vi "FPGA Co-Wound Test.vi"() -> ()   [LabVIEW 2018]
doc: "Author: Scott Hannahs <sth@magnet.fsu.edu>\nCopyright 2018 Florida State University, All rights reserved."
uses:
  <vilib>/eio/EIONode/EIONode.xnode
  <vilib>/rvi/eio/common/nirviEmuTemplateMethod_errors.vi
  SCH Data Controls/Digitizer State Enum.ctl
  SCH Data Controls/SCH Data 2 RT.ctl
  SCH Data Controls/SCH Int Data with Pressure.ctl
  SCH Data Controls/SCH Raw Int Data.ctl
  <vilib>/rvi/FXPMathLib/FxpInterpret/XNode/nifxpmath_Interpret.xnode
  <vilib>/rvi/DataTransferAndStorage/Container/XNode/niFpgaContainer.xnode
  <vilib>/rvi/interface/RandomDataEmulation/nirviRandomDataFpgaReadWriteTemplate.vi
  <vilib>/rvi/FIFO/Fifo_Resource/nirvififoEmulationWrite.vi
  SCH Scaling Controls/SCH Pressure Offset.ctl
  SCH Scaling Controls/SCH Pressure Offset Array.ctl
  SCH Scaling Controls/SCH Dump Resistor Scale Factor.ctl
  SCH Scaling Controls/SCH Joint Scale Factor.ctl
  SCH Scaling Controls/SCH Joint Scale Factor Array.ctl
  SCH Scaling Controls/SCH SC Bus Scale Factor.ctl
  SCH Scaling Controls/SCH SC Bus Scale Factor Array.ctl
  SCH Scaling Controls/SCH CoWound Scale Factor.ctl
  SCH Scaling Controls/SCH Scale Factor.ctl
  SCH Scaling Controls/SCH Scale Factor Array.ctl
  SCH Data Controls/SCH Data 2 RT Array.ctl
  Init Coil Calibration/FPGA Magnet Config.ctl
panel:
  in  "Magnet Configuration Data":T1={"#Coils"=4, "Coil Inductances"=[0.10000002384185791, 0.3999999761581421, 0.6000000238418579, 1.199999988079071], "Max Coil Currents"=[19.899999976158142, 19.899999976158142, 19.899999976158142, 19.899999976158142], "Max Coil Volt Dev"=[1.800000011920929, 2.100000023841858, 3.100000023841858, 2.600000023841858], "Coil A Coefficients"=[0.8209999799728394, 0.00010001659393310547, 5.960464477539063e-08], "Coil B Coefficients"=[0.8999999761581421, 0.00019997358322143555, 2.9802322387695312e-06], "Coil C Coefficients"=[1.100000023841858, 0.0, 0.0], "Coil D Coefficients"=[1.0, 0.0009999871253967285, 0.0], "Max Coil Temp"=[100.0, 80.0, 80.0, 60.0], " Pressure Range"=[29.30000001192093, 32.30000001192093], "Temp Coef"=[0.0031999945640563965, 0.0031999945640563965, 0.0029000043869018555, 0.004100024700164795], "Offsets"=[0.0, 0.0, -5.0, -5.0, 0.0, 0.0, 0.0, 0.0, 0.0, 0.0, 0.0, 0.0, 0.0, 0.0, 0.0], "Scale Factors"=[20.0, 20.0, 4.2670000195503235, 4.269999980926514, 2.0, 1.0, 1.0, 1.0, 1.0, 1.0, -2.0, 30.08600002527237, 29.861999988555908, 35.50199997425079, 35.56999999284744]} {"Coil D Coefficients" format="%_6g"; "Coil C Coefficients" format="%_6g"; "Coil B Coefficients" format="%_6g"; "Scale Factors" format="%_5g"; "Offsets" format="%_5g"; "Temp Coef" format="%_6g"; "Max Coil Temp" format="%_6g"; "Max Coil Volt Dev" format="%_6g"; "Max Coil Currents" format="%_6g"; "Coil Inductances" format="%_6g"; "Pressure Range" format="%_6g"; "Coil A Coefficients" format="%_6g"}
  in  "Input Select":T3(ring)
  in  "Inject frequency (Hz)":fxp<+,32,16>
  in  "Inject Offset":fxp<+/-,16,5> format="%.3g"
  in  "Inject Channel":i32=1
  out "Scale":T4
  out "Calibrate Index":i16
  out "Offset":T4
  out "Main Index":i32
  in  "Reset":bool
  out "DAQ Loop WDT":bool
  out "Filt Data":T5=[0.0, 0.0, 0.0, 0.0, 0.0, 0.0, 0.0, 0.0, 0.0, 0.0, 0.0, 0.0, 0.0, 0.0, 0.0, 0.0, 0.0, 0.0, 0.0, 0.0, 0.0, 0.0, 0.0, 0.0, 0.0, 0.0, 0.0, 0.0, 0.0, 0.0, 0.0, 0.9999999701976776, 0.0, 0.0, -1.0, 0.9999999701976776, -1.0, -1.0, 0.9971923828125, 0.0, 0.0, 0.0, 0.0, 0.0, 0.0, -1.0, 0.0, 0.0, 0.0, 0.0, 0.0, 0.0, 0.0, 0.0] format="%_6g"
  out "Filt Data 2":T5 format="%_6g"
  in  "Layer Scale Factors":T6=[3.0, 3.0, 3.0, 3.0, 3.0, 3.0, 3.0, 3.0, 3.0, 3.0, 3.0, 3.0, 3.0, 3.0, 3.0, 3.0, 3.0, 3.0]
  in  "Co-Wound Scale Factor":T8=200.0
  in  "SC Bus Scale":T9=[0.0009765326976776123, 0.0009765326976776123, 0.0009765326976776123, 0.0009765326976776123, 0.0009765326976776123, 0.0009765326976776123]
  in  "Joint Scale Factors":T11=[1.0013580322265625e-05, 1.0013580322265625e-05, 1.0013580322265625e-05, 1.0013580322265625e-05, 1.0013580322265625e-05, 1.0013580322265625e-05, 1.0013580322265625e-05, 1.0013580322265625e-05]
  in  "DAQ Cycle Ticks":u32=4096
  out "uSec/Cycle":u32
  in  "Ln2 Filter Size":i16=10
  in  "Dump Resistor Scale Factor":T13=200.0
  out "Dump Resistor Voltage":T2 format="%_6g"
  in  "Pressure Offsets":T14=[-8.5, -8.5]
  out "Data Size":i32
  out "Timed Out? FIFO2RT Filter":bool
  out "Timed Out? FIFO Raw":bool
  in  "Pressure Scale Factor":T2[](array[typedef])=[1.723690003156662, 1.723690003156662, 1.723690003156662, 1.723690003156662] format="%_6g"
  in  "stop 2":bool
  out "Timed Out? FIFO2RT Raw":bool
  in  "stop":bool
  # "mH"
  # "kA"
  # "V"
  # "mOhm"
  # "mOhm"
  # "mOhm"
  # "mOhm"
  # "Deg C"
  # "bar"
  # "1/Deg C"
  # "Tin"
  # "Tout"
  # "Pin"
  # "Pout"
  # "I"
  # "WDTin"
  # "PSEnb"
  # "CellFLT"
  # "WDTout"
  # "BTFlt"
  # "BTvolt"
  # "Va"
  # "Vb"
  # "Vc"
  # "Vd"
  # "Tin"
  # "Tout"
  # "Pin"
  # "Pout"
  # "I"
  # "WDTin"
  # "PSEnb"
  # "CellFLT"
  # "WDTout"
  # "BTFlt"
  # "BTvolt"
  # "Va"
  # "Vb"
  # "Vc"
  # "Vd"
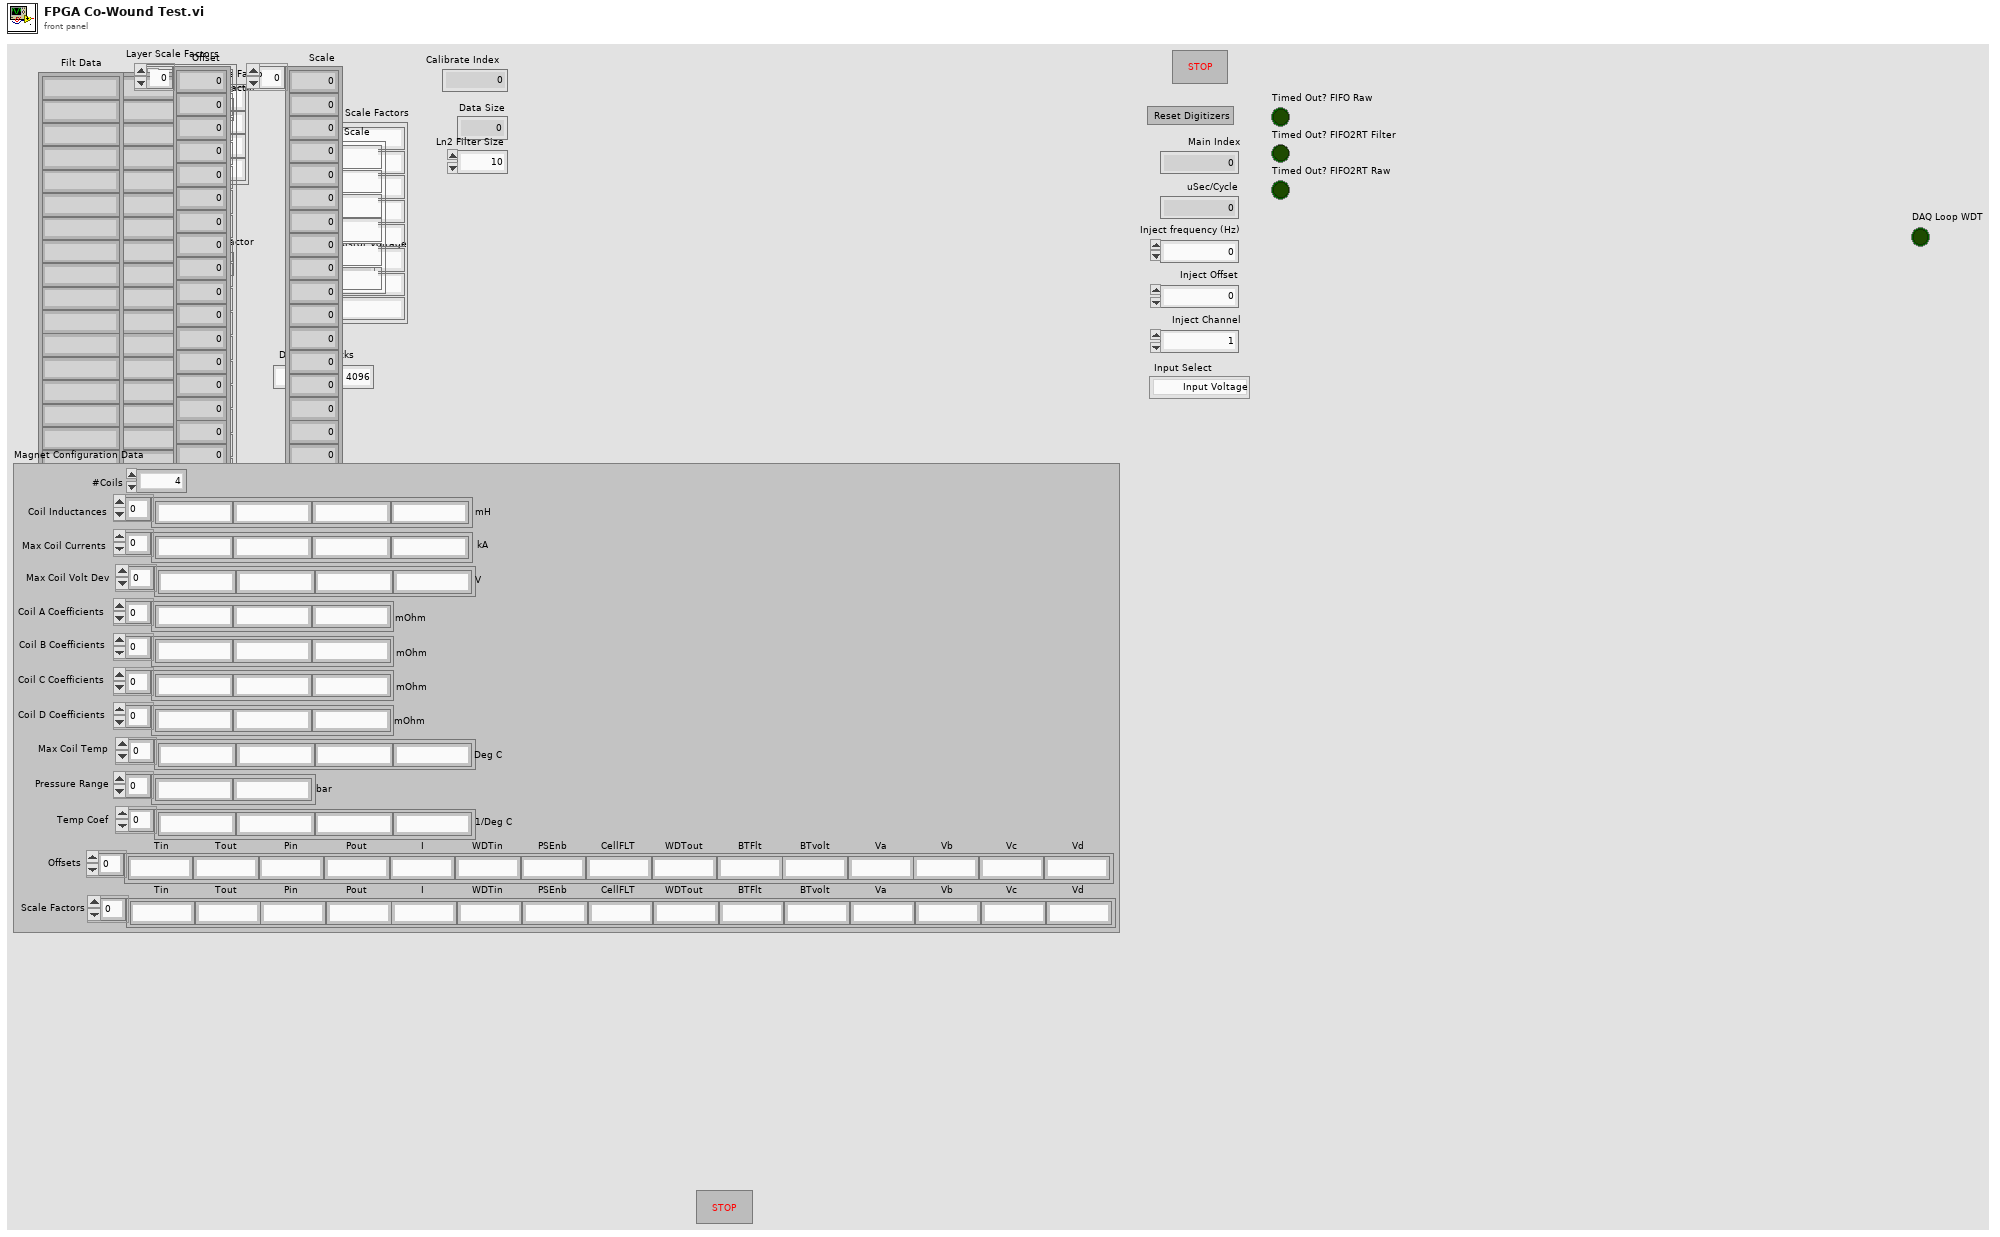
[diagram p1: front panel]
types:
  T1 = typedef "FPGA Magnet Config.ctl" = cluster{"#Coils":u32, "Coil Inductances":T2[], "Max Coil Currents":T2[], "Max Coil Volt Dev":T2[], "Coil A Coefficients":T2[], "Coil B Coefficients":T2[], "Coil C Coefficients":T2[], "Coil D Coefficients":T2[], "Max Coil Temp":T2[], " Pressure Range":T2[], "Temp Coef":T2[], "Offsets":T2[], "Scale Factors":T2[]}
  T2 = typedef "SCH Data 2 RT.ctl" = fxp<+/-,38,12>
  T3 = enum16{"Input Voltage", "Zero Voltage", "Calibrate Voltage"}
  T4 = typedef "SCH Raw Int Data.ctl" = i16[]
  T5 = typedef "SCH Data 2 RT Array.ctl" = T2[]
  T6 = typedef "SCH Scale Factor Array.ctl" = T7[]
  T7 = typedef "SCH Scale Factor.ctl" = fxp<+/-,16,6>
  T8 = typedef "SCH CoWound Scale Factor.ctl" = fxp<+/-,16,12>
  T9 = typedef "SCH SC Bus Scale Factor Array.ctl" = T10[]
  T10 = typedef "SCH SC Bus Scale Factor.ctl" = fxp<+/-,38,12>
  T11 = typedef "SCH Joint Scale Factor Array.ctl" = T12[]
  T12 = typedef "SCH Joint Scale Factor.ctl" = fxp<+/-,38,12>
  T13 = typedef "SCH Dump Resistor Scale Factor.ctl" = fxp<+/-,16,12>
  T14 = typedef "SCH Pressure Offset Array.ctl" = T15[]
  T15 = typedef "SCH Pressure Offset.ctl" = fxp<+/-,16,5>
  T16 = typedef "Digitizer State Enum.ctl" = enum16{"Reset", "StartCnvt"}
  T17 = typedef "SCH Int Data with Pressure.ctl" = fxp<+/-,19,5>[]
  T18 = typedef "SCH All FXP Data.ctl" = fxp<+/-,19,5>[]
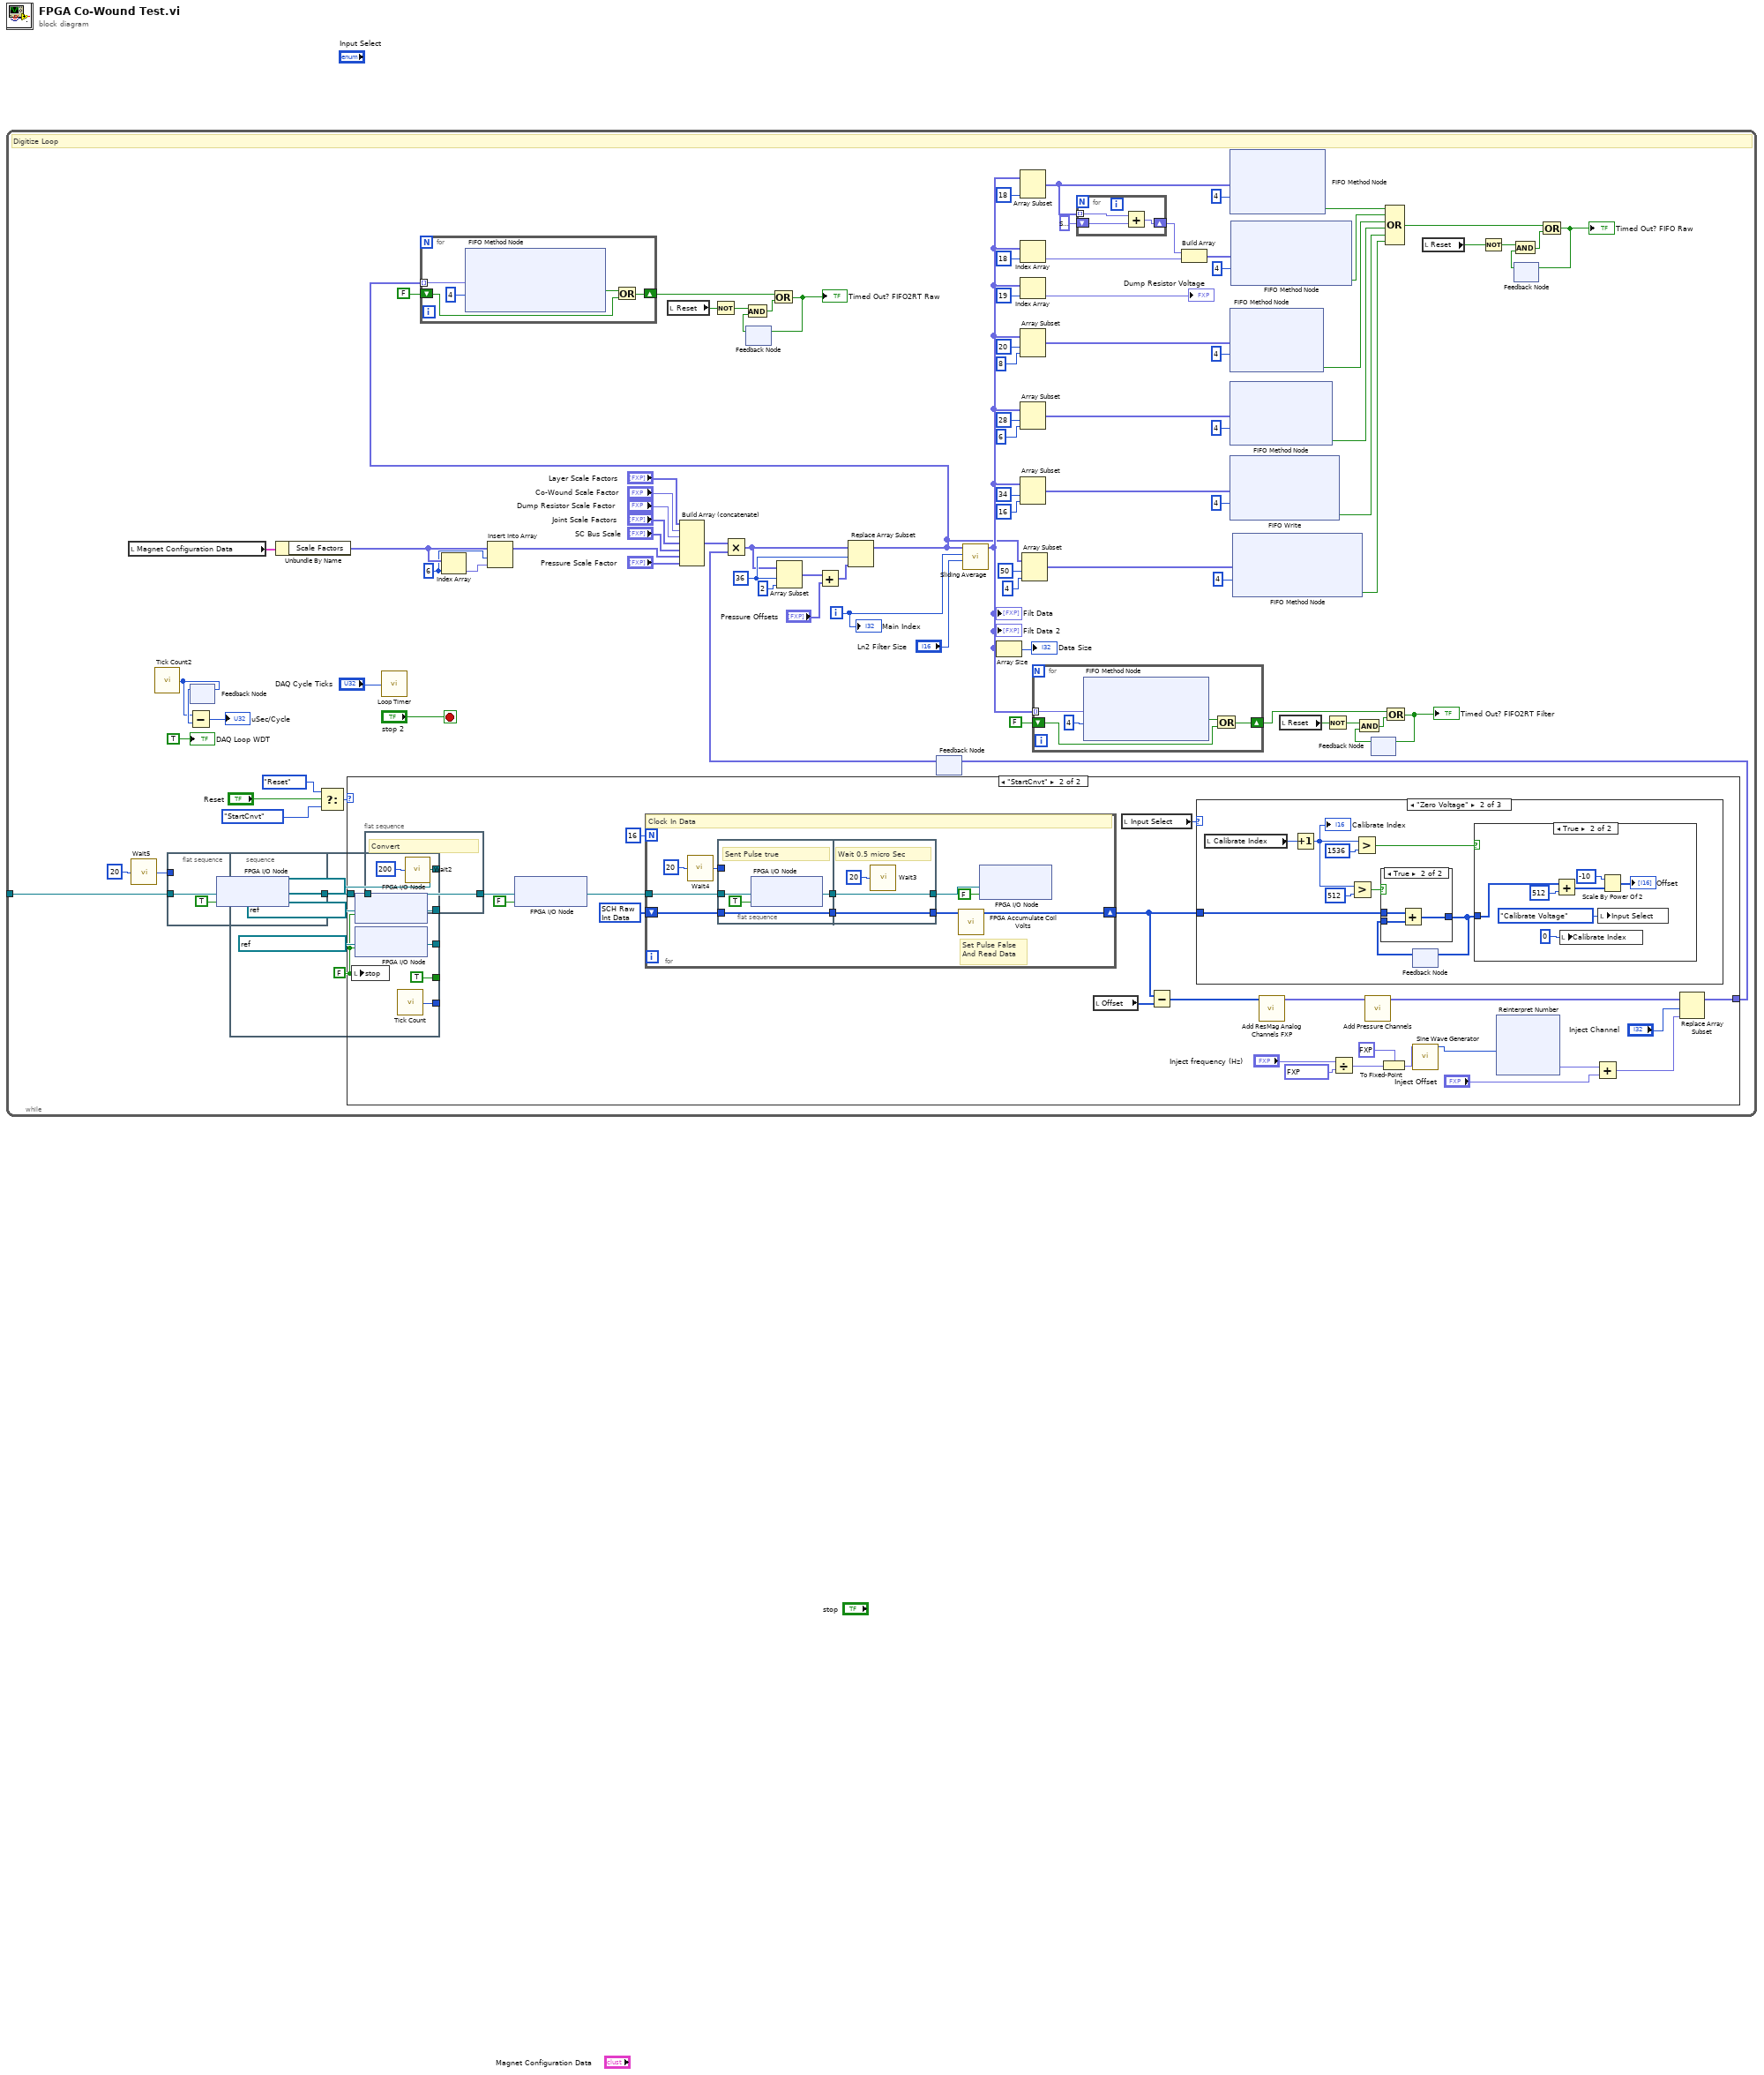
[diagram p0: block diagram]
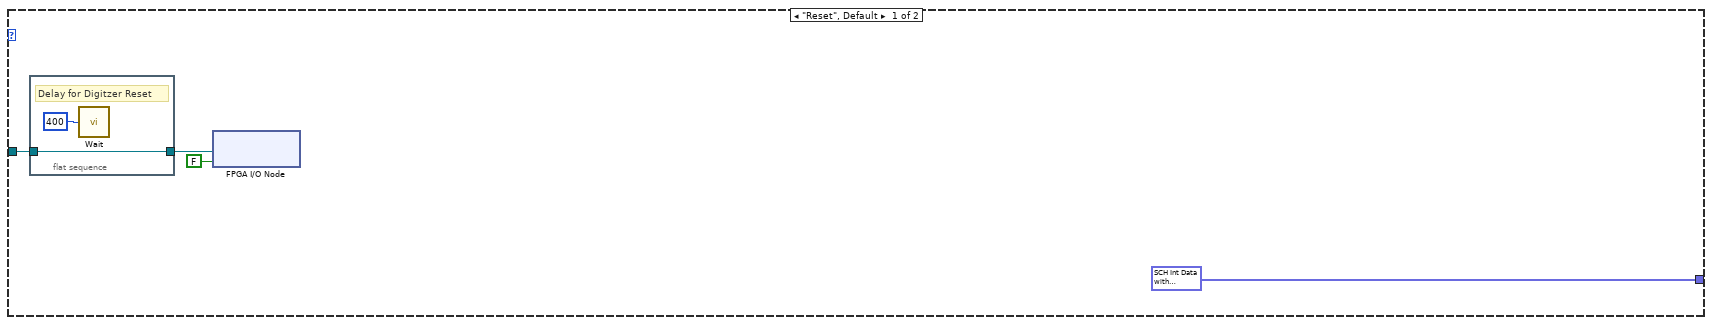
[diagram p2: hidden frame]
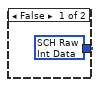
[diagram p5: hidden frame]
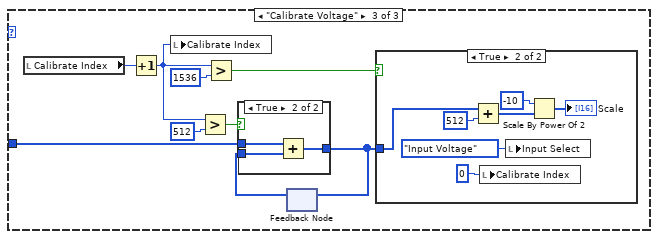
[diagram p6: hidden frame]
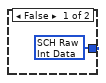
[diagram p8: hidden frame]
diagram:
  n1 = while {
    tunnel: _ -> [w87]
    i -> [w58]
    stop <- "stop 2" stop-if-true
    w29 = 6 ("index")
    w62 = 36 ("index")
    # "Digitize Loop"
    n2 = local read "Magnet Configuration Data"() -> (w76:T1)
    n3 = call "Wait5"("Count(Ticks)"=u32 20 ("Count(uSec)")) -> ("Tick Count(Ticks)"=w88:u32)
    n4 = call "Tick Count2"() -> ("Tick Count(uSec)"=w71:u32)
    n5 = flat-sequence {
      tunnel: w88 -> [_]
      tunnel: w87 -> [w107]
      tunnel: [w106] -> w86
      frame #0 {
        n6 = xnode "FPGA I/O Node"("I/O Item"=TRUE ("Connector0/DIO0"), "FPGA I/O In"=w107) -> ("FPGA I/O Out"=w106:refnum<k21>)
      }
    }
    n7 = feedback #1() -> (w72:u32)  [unwired: 1 in]
    n8 = Subtract(x=w71, y=w72) -> (x-y=→"uSec/Cycle":u32)
    n9 = feedback-in #1(w71) -> ()
    n10 = Unbundle By Name(w76) -> ("Scale Factors"=w30:T2[])
    n11 = Select(t=Digitizer_State_Enum."Reset", s="Reset", f=Digitizer_State_Enum."StartCnvt" ("t")) -> (s? t:f=w90:T16)
    n12 = case shown="\"StartCnvt\"" w90 {
      tunnel: w86 -> [w110 w135]
      tunnel: [T17 [0.0, 0.0, 0.0, 0.0, 0.0, 0.0, 0.0, 0.0, 0.0, 0.0, 0.0, 0.0, 0.0, 0.0, 0.0, 0.0, 0.0, 0.0, 0.0, 0.0, 0.0, 0.0, 0.0, 0.0, 0.0, 0.0, 0.0, 0.0, 0.0, 0.0, 0.0, 0.0, 0.0, 0.0, 0.0, 0.0, 0.0, 0.0, 0.0, 0.0, 0.0, 0.0, 0.0, 0.0, 0.0, 0.0, 0.0, 0.0, 0.0, 0.0, 0.0, 0.0, 0.0, 0.0] ("Array") w130] -> w73
      frame "Reset", Default {
        n13 = flat-sequence {
          tunnel: [w114] -> w111
          tunnel: w110 -> [w114]
          frame #0 {
            # "Delay for Digitzer Reset"
            n14 = call "Wait"("Count(Ticks)"=u32 400 ("Count(uSec)")) -> ()  [unwired: 1 out]
          }
        }
        n15 = xnode "FPGA I/O Node"("I/O Item"=FALSE ("Connector0/DIO0"), "FPGA I/O In"=w111) -> ()  [unwired: 1 out]
      }
      frame "StartCnvt" {
        n16 = flat-sequence {
          tunnel: [w195] -> w134
          tunnel: w135 -> [w195]
          frame #0 {
            # "Convert"
            n17 = call "Wait2"("Count(Ticks)"=u32 200 ("Count(uSec)")) -> ()  [unwired: 1 out]
          }
        }
        n18 = xnode "FPGA I/O Node"("I/O Item"=FALSE ("Connector0/DIO0"), "FPGA I/O In"=w134) -> ("FPGA I/O Out"=w136:refnum<k21>)
        n19 = for {
          N: 16 -> [_]
          shift-right: [w178] -> w115
          shift-left: T4 [0, 0, 0, 0, 0, 0, 0, 0, 0, 0, 0, 0, 0, 0, 0, 0, 0, 0, 0, 0, 0, 0, 0, 0, 0, 0, 0, 0, 0, 0, 0, 0, 0, 0, 0, 0, 0, 0] -> [w181]
          tunnel: w136 -> [w182]
          # "Set Pulse False\nAnd Read Data"
          # "Clock In Data"
          n20 = call "Wait4"("Count(Ticks)"=u32 20 ("Count(uSec)")) -> ("Tick Count(Ticks)"=w185:u32)
          n21 = flat-sequence {
            tunnel: w185 -> [_]
            tunnel: w182 -> [w190]
            tunnel: [w189] -> w187
            tunnel: w181 -> [w188]
            tunnel: [w188] -> w180
            tunnel: [w194] -> w184
            tunnel: w187 -> [w194]
            tunnel: [w192] -> w179
            tunnel: w180 -> [w192]
            frame #0 {
              # "Sent Pulse true"
              n22 = xnode "FPGA I/O Node"("I/O Item"=TRUE ("Connector0/DIO0"), "FPGA I/O In"=w190) -> ("FPGA I/O Out"=w189:refnum<k21>)
            }
            frame #1 {
              # "Wait 0.5 micro Sec"
              n23 = call "Wait3"("Count(Ticks)"=u32 20 ("Count(uSec)")) -> ()  [unwired: 1 out]
            }
          }
          n24 = call "FPGA Accumulate Coil Volts.vi"("Data Array In"=w179) -> ("Data Array Out"=w178:T4)  [unwired: 10 in]
          n25 = xnode "FPGA I/O Node"("I/O Item"=FALSE ("Connector0/DIO0"), "FPGA I/O In"=w184) -> ()  [unwired: 1 in, 2 out]
        }
        n26 = local read "Offset"() -> (w122:T4)
        n27 = local read "Input Select"() -> (w121:T3)
        n28 = Subtract(x=w115, y=w122) -> (x-y=w120:T4)
        n29 = case shown="\"Zero Voltage\"" w121 {
          tunnel: w115 -> [_ w143 w163]
          frame "Input Voltage", Default {
          }
          frame "Zero Voltage" {
            n30 = local read "Calibrate Index"() -> (w145:i16)
            n31 = Increment(x=w145) -> (x+1=w138:i16)
            "Calibrate Index" <- w138
            n32 = Greater?(x=w138, y=i16 512) -> (0:w144:bool)
            n33 = Greater?(x=w138, y=i16 1536) -> (0:w141:bool)
            n34 = feedback #2() -> (w139:i32[])  [unwired: 1 in]
            n35 = case shown="True" w144 {
              tunnel: w143 -> [_ w157]
              tunnel: [T4 [0, 0, 0, 0, 0, 0, 0, 0, 0, 0, 0, 0, 0, 0, 0, 0, 0, 0, 0, 0, 0, 0, 0, 0, 0, 0, 0, 0, 0, 0, 0, 0, 0, 0, 0, 0, 0, 0] ("Scale") w156] -> w140
              tunnel: w139 -> [_ w155]
              frame False {
              }
              frame True {
                n36 = Add(x=w157, y=w155) -> (x+y=w156:i32[])
              }
            }
            n37 = feedback-in #2(w140) -> ()
            n38 = case shown="True" w141 {
              tunnel: w140 -> [_ w152]
              frame False {
              }
              frame True {
                n39 = Add(x=w152, y=512 ("n")) -> (x+y=w148:i32[])
                n40 = local write "Calibrate Index"(i16 0 ("Calibrate Index")) -> ()
                n41 = local write "Input Select"(T3."Calibrate Voltage" ("Input Select")) -> ()
                n42 = Scale By Power Of 2(n=i16 -10, x=w148) -> (x*2^n=→"Offset":i32[])
              }
            }
          }
          frame "Calibrate Voltage" {
            n43 = local read "Calibrate Index"() -> (w165:i16)
            n44 = Increment(x=w165) -> (x+1=w158:i16)
            n45 = local write "Calibrate Index"(w158) -> ()
            n46 = Greater?(x=w158, y=i16 512) -> (0:w164:bool)
            n47 = Greater?(x=w158, y=i16 1536) -> (0:w161:bool)
            n48 = feedback #3() -> (w159:i32[])  [unwired: 1 in]
            n49 = case shown="True" w164 {
              tunnel: w163 -> [_ w177]
              tunnel: [T4 [0, 0, 0, 0, 0, 0, 0, 0, 0, 0, 0, 0, 0, 0, 0, 0, 0, 0, 0, 0, 0, 0, 0, 0, 0, 0, 0, 0, 0, 0, 0, 0, 0, 0, 0, 0, 0, 0] ("Scale") w176] -> w160
              tunnel: w159 -> [_ w175]
              frame False {
              }
              frame True {
                n50 = Add(x=w177, y=w175) -> (x+y=w176:i32[])
              }
            }
            n51 = feedback-in #3(w160) -> ()
            n52 = case shown="True" w161 {
              tunnel: w160 -> [_ w172]
              frame False {
              }
              frame True {
                n53 = Add(x=w172, y=512 ("n")) -> (x+y=w168:i32[])
                n54 = local write "Calibrate Index"(i16 0 ("Calibrate Index")) -> ()
                n55 = local write "Input Select"(T3."Input Voltage" ("Input Select")) -> ()
                n56 = Scale By Power Of 2(n=i16 -10, x=w168) -> (x*2^n=→"Scale":i32[])
              }
            }
          }
        }
        n57 = call "Add ResMag Analog Channels FXP.vi"("Array in"=w120) -> ("Array out"=w123:T18)  [unwired: 10 in]
        n58 = Divide(x="Inject frequency (Hz)", y=fxp<+,32,26> 40000000.0) -> (x/y=w128:fxp<+,64,22>)
        n59 = call "Add Pressure Channels.vi"("Array in"=w123) -> ("Array Out"=w119:T17)  [unwired: 10 in]
        n60 = To Fixed-Point(fixed-point type=fxp<+,32,0> 0.0 ("frequency (periods/tick)"), number=w128) -> (fixed-point=w126:fxp<+,32,0>)
        n61 = call "Sine Wave Generator"("frequency (periods/tick)"=w126) -> ("sine out"=w131:i16)  [unwired: 14 in]
        n62 = xnode "Reinterpret Number"("x"=w131) -> ("y"=w118:fxp<+/-,16,5>)
        n63 = Add(x=w118, y="Inject Offset") -> (x+y=w117:fxp<+/-,19,5>)
        n64 = Replace Array Subset(array=w119, new element=w117, index="Inject Channel") -> (w130:T17)
      }
    }
    n65 = call "Loop Timer"("Count(Ticks)"="DAQ Cycle Ticks") -> ()  [unwired: 1 out]
    n66 = Index Array(array=w30, index=w29) -> (element=w31:T2)
    n67 = Insert Into Array(array=w30, index=w29, new element=w31) -> (w32:T2[])
    n68 = local read "Reset"() -> (w6:bool)
    n69 = Build Array (concatenate)("Layer Scale Factors", "Co-Wound Scale Factor", "Dump Resistor Scale Factor", "Joint Scale Factors", "SC Bus Scale", w32, "Pressure Scale Factor") -> (w64:T2[])
    n70 = Not(x=w6) -> (.not. x?=w7:bool)
    n71 = feedback #4() -> (w4:bool)  [unwired: 1 in]
    n72 = And(x=w7, y=w4) -> (x .and. y?=w5:bool)
    n73 = feedback-in #5(w73) -> ()
    n74 = feedback #5() -> (w33:T17)  [unwired: 1 in]
    n75 = Multiply(x=w64, y=w33) -> (x*y=w28:T2[])
    n76 = Array Subset(array=w28, index=w62, length=2) -> (w61:T2[])
    n77 = Add(x=w61, y="Pressure Offsets") -> (x+y=w60:T2[])
    n78 = Replace Array Subset(array=w28, new element=w60, index=w62) -> (w2:T2[])
    n79 = for {
      tunnel: w2 -> [w97] mode=indexing
      shift-right: [w95] -> w8
      shift-left: FALSE -> [w94]
      n80 = xnode ("FIFO Method Node")("Element"=w97, "Timeout"=4) -> ("Timed Out?"=w96:bool)  [unwired: 1 in, 1 out]
      n81 = Or(x=w96, y=w94) -> (x .or. y?=w95:bool)
    }
    n82 = Or(x=w8, y=w5) -> (x .or. y?=w9:bool)
    "Timed Out? FIFO2RT Raw" <- w9
    n83 = feedback-in #4(w9) -> ()
    n84 = call "Sliding Average.vi"("Ln2 Filter Size"="Ln2 Filter Size", 10:w58, "Array In"=w2) -> ("Filtered Array Out"=w37:T5)  [unwired: 8 in]
    "Filt Data" <- w37
    "Filt Data 2" <- w37
    n85 = Array Size(array=w37) -> (size(s)=→"Data Size":i32)
    n86 = Array Subset(array=w37, length=18) -> (w52:T2[])  [unwired: 1 in]
    n87 = Index Array(array=w37, index=18) -> (element=w49:T2)
    n88 = Index Array(array=w37, index=19) -> (element=→"Dump Resistor Voltage":T2)
    n89 = Array Subset(array=w37, index=20, length=8) -> (w48:T2[])
    n90 = Array Subset(array=w37, index=28, length=6) -> (w47:T2[])
    n91 = Array Subset(array=w37, index=34, length=16) -> (w53:T2[])
    n92 = Array Subset(array=w2, index=50, length=4) -> (w36:T2[])
    n93 = for {
      tunnel: w37 -> [w105] mode=indexing
      shift-right: [w103] -> w17
      shift-left: FALSE -> [w102]
      n94 = xnode ("FIFO Method Node")("Element"=w105, "Timeout"=4) -> ("Timed Out?"=w104:bool)  [unwired: 1 in, 1 out]
      n95 = Or(x=w104, y=w102) -> (x .or. y?=w103:bool)
    }
    n96 = for {
      tunnel: w52 -> [w99] mode=indexing
      shift-right: [w98] -> w50
      shift-left: T2 0.0 ("Numeric") -> [w100]
      n97 = Add(x=w99, y=w100) -> (x+y=w98:T2)
    }
    n98 = Build Array(w50, w49) -> (w82:T2[])
    n99 = xnode ("FIFO Method Node")("Element"=w52, "Timeout"=4) -> ("Timed Out?"=w42:bool)  [unwired: 1 in, 1 out]
    n100 = xnode ("FIFO Method Node")("Element"=w48, "Timeout"=4) -> ("Timed Out?"=w25:bool)  [unwired: 1 in, 1 out]
    n101 = xnode ("FIFO Method Node")("Element"=w47, "Timeout"=4) -> ("Timed Out?"=w24:bool)  [unwired: 1 in, 1 out]
    n102 = xnode ("FIFO Write")("Element"=w53, "Timeout"=4) -> ("Timed Out?"=w23:bool)  [unwired: 1 in, 1 out]
    n103 = xnode ("FIFO Method Node")("Element"=w82, "Timeout"=4) -> ("Timed Out?"=w26:bool)  [unwired: 1 in, 1 out]
    n104 = xnode ("FIFO Method Node")("Element"=w36, "Timeout"=4) -> ("Timed Out?"=w22:bool)  [unwired: 1 in, 1 out]
    n105 = local read "Reset"() -> (w19:bool)
    n106 = Not(x=w19) -> (.not. x?=w18:bool)
    n107 = feedback #6() -> (w21:bool)  [unwired: 1 in]
    n108 = And(x=w18, y=w21) -> (x .and. y?=w20:bool)
    n109 = Or(x=w17, y=w20) -> (x .or. y?=w16:bool)
    "Timed Out? FIFO2RT Filter" <- w16
    n110 = feedback-in #6(w16) -> ()
    n111 = Compound Arithmetic op=OR(w42, w26, w25, w24, w23, w22) -> (w11:bool)
    n112 = local read "Reset"() -> (w13:bool)
    n113 = Not(x=w13) -> (.not. x?=w12:bool)
    n114 = feedback #7() -> (w15:bool)  [unwired: 1 in]
    n115 = And(x=w12, y=w15) -> (x .and. y?=w14:bool)
    n116 = Or(x=w11, y=w14) -> (x .or. y?=w10:bool)
    "Timed Out? FIFO Raw" <- w10
    n117 = feedback-in #7(w10) -> ()
    "Main Index" <- w58
    "DAQ Loop WDT" <- TRUE ("DAQ Loop WDT")
  }
  n118 = stacked-sequence {
    tunnel: [w204] -> _
    tunnel: [TRUE] -> _
    tunnel: [w201] -> _
    tunnel: [w198] -> _
    tunnel: [refnum<k21> "Digitizer Read Error" ("FPGA I/O In")] -> _
    frame #0 {
      w199 = FALSE ("Connector0/DIO0")
      n119 = local write "stop"(w199) -> ()
      n120 = xnode "FPGA I/O Node"("I/O Item"=w199, "FPGA I/O In"=refnum<k21> "Digitizer Calibrate") -> ("FPGA I/O Out"=w198:refnum<k21>)
      n121 = xnode "FPGA I/O Node"("I/O Item"=w199, "FPGA I/O In"=refnum<k21> "Digitizer Clock Data") -> ("FPGA I/O Out"=w204:refnum<k21>)
      n122 = call "Tick Count"() -> ("Tick Count(Ticks)"=w201:u32)
    }
  }
